vi "Write I vs nm Graph Ref.vi"(8 "error in (no error)":errorcluster, 10 "I vs nm Graph Ref":refnum<vi>, 11 "Analyze Results FF-Spectrum in":refnum<class "Analyze Results FF-Spectrum.lvclass">) -> (0 "error out":errorcluster, 3 "Analyze Results FF-Spectrum out":refnum<class "Analyze Results FF-Spectrum.lvclass">)   [LabVIEW 2014, in "Analyze Results FF-Spectrum.lvclass"]
uses:
  Analyze Results FF-Spectrum.lvclass
  Analyze Results FF-Spectrum.lvclass/Analyze Results FF-Spectrum.ctl
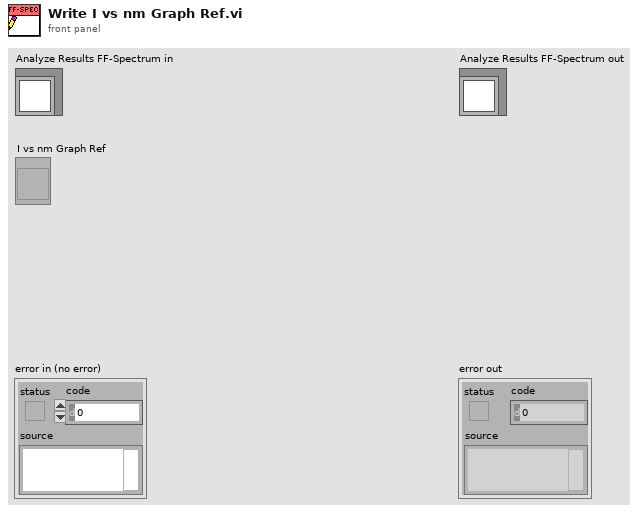
[diagram p1: front panel]
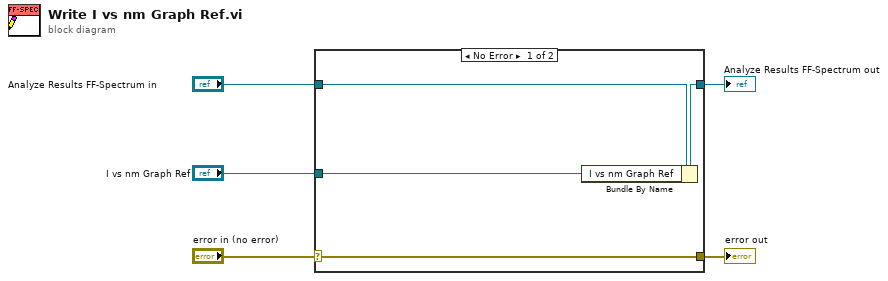
[diagram p0: block diagram]
diagram:
  n1 = case shown="No Error" "error in (no error)" {
    selector: "error in (no error)" -> [w9 w10]
    tunnel: [w9 w10] -> w4
    tunnel: [w7 w11] -> w2
    tunnel: "Analyze Results FF-Spectrum in" -> [w8 w11]
    tunnel: "I vs nm Graph Ref" -> [w6 _]
    frame No Error {
      n2 = Bundle By Name(cluster=w8, "I vs nm Graph Ref"=w6) -> (w7:refnum<class "Analyze Results FF-Spectrum.lvclass">)
    }
    frame Error {
    }
  }
  "error out" <- w4
  "Analyze Results FF-Spectrum out" <- w2
